vi "Audio Test.vi"() -> ()   [LabVIEW 2020, in "obs-scratch.lvlib"]
uses:
  obs-scratch.lvlib
  g-audio/src/LabVIEW/G-Audio/Controls/Audio Device Config.ctl
  g-audio/src/LabVIEW/G-Audio/Controls/Audio Device Format.ctl
  g-audio/src/LabVIEW/G-Audio/Controls/Backends.ctl
  g-audio/src/LabVIEW/G-Audio/Controls/Audio Device Info.ctl
  g-audio/src/LabVIEW/G-Audio/Controls/Audio Device Type.ctl
  g-audio/src/LabVIEW/G-Audio/Controls/Audio Device Native Data Format.ctl
  93cf9091-5c46-455b-b0da-0cb22890f002.vi
  <vilib>/Analysis/5stat.llb/RMS (DBL).vi
  g-audio/src/LabVIEW/G-Audio/Private/Result To Error.vi
  93cf9091-5c46-455b-b0da-0cb22890f002.vi/6b901882-6109-4f44-aca5-48e1525e5248.vi
  93cf9091-5c46-455b-b0da-0cb22890f002.vi/06c0137a-63d3-4e30-982f-115d83a1188c.vi
  g-audio/src/LabVIEW/G-Audio/Audio Devices/Get Audio Device Configuration.vi
  g-audio/src/LabVIEW/G-Audio/Private/Audio Device Refnum To Value.vi
  93cf9091-5c46-455b-b0da-0cb22890f002.vi/06c0137a-63d3-4e30-982f-115d83a1188c.vi/4b7b629c-2e91-4160-9820-a26af8f6e677.vi
  g-audio/src/LabVIEW/G-Audio/Private/ma_format To Audio Data Format.vi
  <vilib>/Utility/Data Type/Get Numeric Information.vi
  <vilib>/Utility/error.llb/Error Cluster From Error Code.vi
  g-audio/src/LabVIEW/G-Audio/G-Audio.lvlib
  <vilib>/Analysis/NI_AALPro.lvlib
  obs-websocket/OBS/OBS.lvclass
panel:
  in  "Gain":dbl
  in  "Scale Decay":dbl(slide) scale=0.0..1.0
  out "Scale":dbl(knob) scale=0.8..1.2
  in  "Password":string="44S4aN6PpCHpVM4Y"
  out "Meter":dbl(knob) scale=0.8..1.2
  out "error out":errorcluster
  in  "stop":bool
  out "Waveform":waveform(dbl)[](graph)
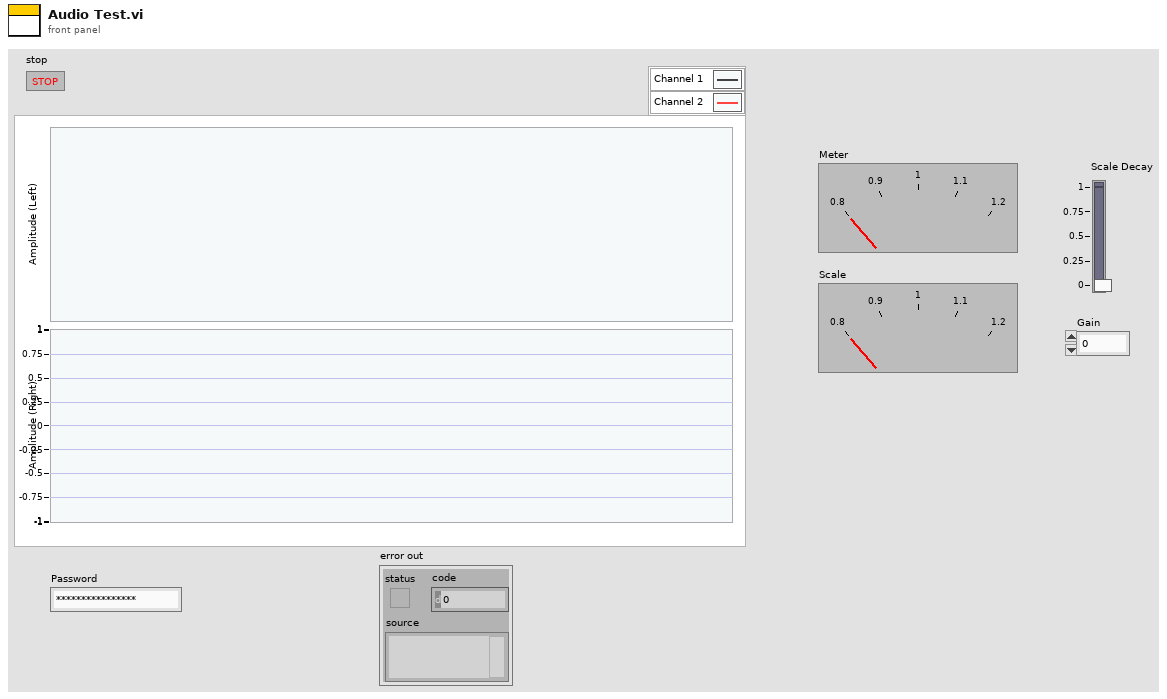
[diagram p1: front panel]
types:
  T1 = typedef "G-Audio.lvlib/Audio Device Type.ctl" = enum16{"(None)", "Playback", "Capture", "Duplex", "Loopback"}
  T2 = typedef "G-Audio.lvlib/Audio Device Info.ctl" = cluster{"Name":string, "ID":u8[], "Device Type":T1, "Default":bool, "Native Data Formats":T3[]}
  T3 = typedef "G-Audio.lvlib/Audio Device Native Data Format.ctl" = cluster{"Format":T4, "Channels":u32, "Sample Rate (Hz)":u32, "Exclusive Mode":bool}
  T4 = typedef "G-Audio.lvlib/Audio Device Format.ctl" = enum16{"Native", "U8", "I16", "I32", "SGL"}
  T5 = typedef "G-Audio.lvlib/Backends.ctl" = enum16{"WASAPI", "DirectSound", "WinMM", "Core Audio", "sndio", "audio(4)", "OSS", "PulseAudio", "ALSA", "JACK", "AAudio", "OpenSL|ES", "Web Audio", "Custom", "Null", "Default"}
  T6 = typedef "G-Audio.lvlib/Audio Device Config.ctl" = cluster{"Sample Rate (Hz)":u32, "Channels":u32, "Format":T4}
  T7 = typedef "G-Audio.lvlib/Audio Device Refnum.ctl" = refnum<file>
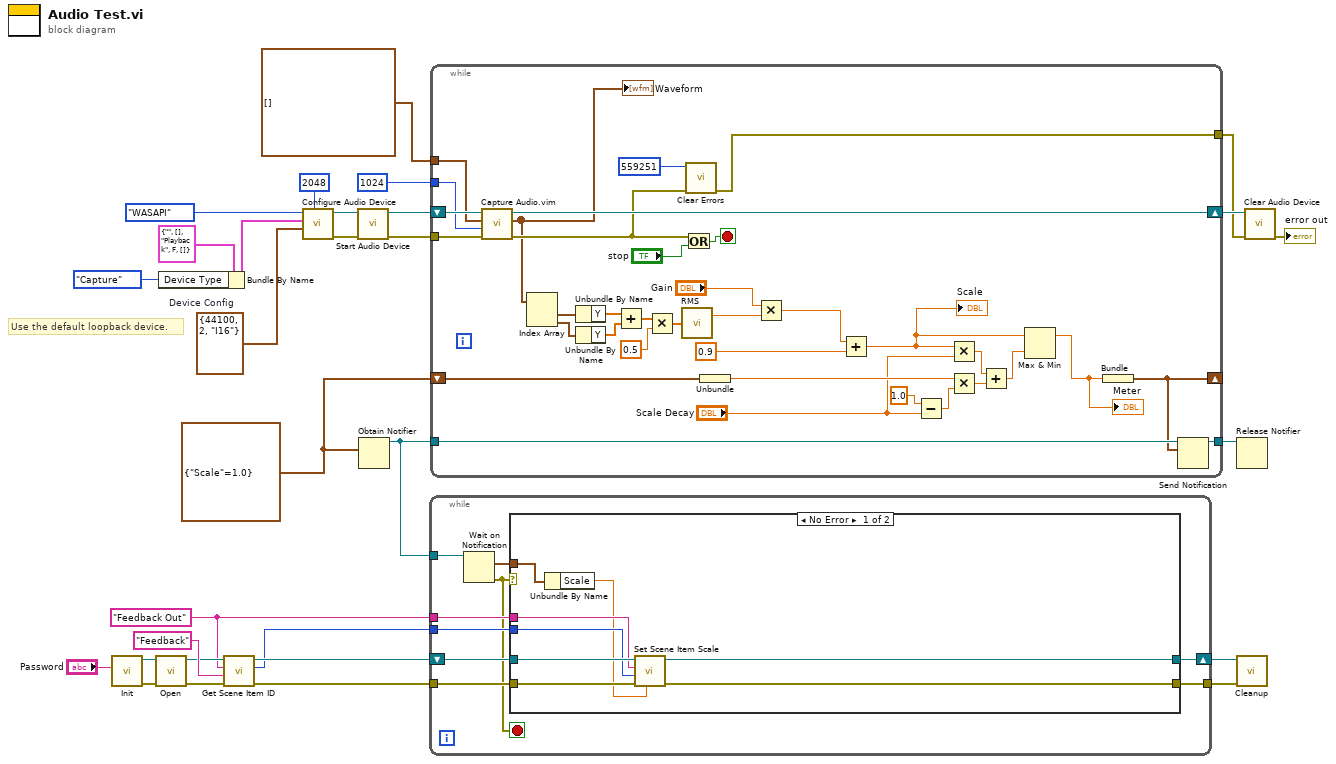
[diagram p0: block diagram]
diagram:
  w1 = cluster{"Scale":dbl} {"Scale"=1.0}
  w5 = "Feedback Out" ("Scene Name")
  w27 = T6 {"Sample Rate (Hz)"=44100, "Channels"=2, "Format"=enum."I16"}  # Device Config
  # "Use the default loopback device."
  n1 = call "Init.vi"("Password (None)"="Password") -> ("error out"=w14:errorcluster, "OBS out"=w15:refnum<class "OBS.lvclass">)  [unwired: 9 in]
  n2 = call "Open.vi"("error in (no error)"=w14, "OBS in"=w15) -> ("error out"=w10:errorcluster, "OBS out"=w11:refnum<class "OBS.lvclass">)  [unwired: 8 in]
  n3 = Bundle By Name(cluster=T2 {"Name"="", "ID"=[], "Device Type"=enum."Playback", "Default"=FALSE, "Native Data Formats"=[]} ("Audio Device"), "Device Type"=Audio_Device_Type."Capture") -> (w23:T2)
  n4 = call "Get Scene Item ID.vi"("error in (no error)"=w10, "Source Name"="Feedback" ("Scene Name"), "Scene Name"=w5, "OBS in"=w11) -> ("error out"=w9:errorcluster, "Scene Item ID"=w4:i32, "OBS out"=w8:refnum<class "OBS.lvclass">)  [unwired: 5 in]
  n5 = call "Configure Audio Device.vi"("Buffer Size (4096)"=2048 ("number of samples/ch"), "Device Config"=w27, "Audio Device"=w23, "Backend (Default)"=Backends."WASAPI") -> ("error out"=w30:errorcluster, "Audio Device Refnum"=w29:T7)  [unwired: 4 in, 2 out]
  n6 = call "Start Audio Device.vi"("error in (no error)"=w30, "Audio Device Refnum In"=w29) -> ("error out"=w22:errorcluster, "Audio Device Refnum Out"=w20:T7)  [unwired: 8 in]
  n7 = Obtain Notifier(notification data type=w1) -> (notifier out=w3:refnum<notifier>)  [unwired: 3 in, 2 out]
  n8 = while {
    tunnel: w9 -> [w36]
    shift-right: [w38] -> w7
    shift-left: w8 -> [w39]
    tunnel: [w37] -> w6
    tunnel: w5 -> [w35]
    tunnel: w4 -> [w34]
    tunnel: w3 -> [w33]
    stop <- w32 stop-if-true
    n9 = Wait on Notification(notifier=w33) -> (notification=w31:cluster{"Scale":dbl}, error out=w32:errorcluster)  [unwired: 3 in, 2 out]
    n10 = case shown="No Error" w32 {
      tunnel: w39 -> [w47 w49]
      tunnel: [w46 w49] -> w38
      tunnel: [w45 w48] -> w37
      tunnel: w36 -> [w44 w48]
      tunnel: w35 -> [w43 _]
      tunnel: w34 -> [w42 _]
      tunnel: w31 -> [w41 _]
      frame No Error {
        n11 = Unbundle By Name(w41) -> ("Scale"=w40:dbl)
        n12 = call "Set Scene Item Scale.vi"("Scale"=w40, "error in (no error)"=w44, "Scene Item ID"=w42, "Scene Name"=w43, "OBS in"=w47) -> ("error out"=w45:errorcluster, "OBS out"=w46:refnum<class "OBS.lvclass">)  [unwired: 5 in]
      }
      frame Error {
      }
    }
  }
  n13 = while {
    shift-right: [w83] -> w19
    shift-left: w20 -> [w84]
    tunnel: w22 -> [w81]
    tunnel: [w80] -> w18
    tunnel: 1024 ("number of samples/ch") -> [w75]
    tunnel: waveform(dbl)[] [] -> [w82]
    tunnel: w3 -> [w64]
    tunnel: [w63] -> w2
    shift-right: [w55] -> _
    shift-left: w1 -> [w62]
    stop <- w77 stop-if-true
    n14 = call "Capture Audio.vim"("error in (no error)"=w81, "Samples To Read"=w75, "Data Format"=w82, "Audio Device Refnum In"=w84) -> ("error out"=w78:errorcluster, "Audio Data"=w74:waveform(dbl)[], "Audio Device Refnum Out"=w83:T7)  [unwired: 5 in]
    "Waveform" <- w74
    n15 = Index Array(array=w74) -> (element #1=w73:waveform(dbl), element #2=w72:waveform(dbl))  [unwired: 2 in]
    n16 = Unbundle By Name(w73) -> ("Y"=w71:dbl[])
    n17 = Unbundle By Name(w72) -> ("Y"=w70:dbl[])
    n18 = Add(x=w71, y=w70) -> (x+y=w69:dbl[])
    n19 = Multiply(x=w69, y=0.5) -> (x*y=w67:dbl[])
    n20 = call-poly <vilib>:"RMS.vi"("X"=w67) -> ("rms value"=w66:dbl)  [unwired: 1 out]
    n21 = Or(x=w78, y="stop") -> (x .or. y?=w77:bool)
    n22 = call <vilib>:"Clear Errors.vi"("error in (no error)"=w78, "specific error code to clear (0: all)"=559251) -> ("error out"=w80:errorcluster)  [unwired: 4 in, 1 out]
    n23 = Unbundle(w62) -> ("Scale"=w60:dbl)
    n24 = Multiply(x="Gain", y=w66) -> (x*y=w51:dbl)
    n25 = Add(x=w51, y=0.9) -> (x+y=w54:dbl)
    "Scale" <- w54
    n26 = Subtract(x=1.0, y="Scale Decay") -> (x-y=w59:dbl)
    n27 = Multiply(x=w54, y="Scale Decay") -> (x*y=w56:dbl)
    n28 = Multiply(x=w60, y=w59) -> (x*y=w57:dbl)
    n29 = Add(x=w56, y=w57) -> (x+y=w53:dbl)
    n30 = Max & Min(x=w54, y=w53) -> (max(x,y)=w52:dbl)  [unwired: 1 out]
    "Meter" <- w52
    n31 = Bundle(w52) -> (w55:cluster{dbl})  [unwired: 1 in]
    n32 = Send Notification(notification=w55, notifier=w64) -> (notifier out=w63:refnum<notifier>)  [unwired: 1 in, 1 out]
  }
  n33 = Release Notifier(notifier=w2) -> ()  [unwired: 2 in, 3 out]
  n34 = call "Cleanup.vi"("error in (no error)"=w6, "OBS in"=w7) -> ()  [unwired: 9 in, 1 out]
  n35 = call "Clear Audio Device.vi"("error in (no error)"=w18, "Audio Device Refnum In"=w19) -> ("error out"=→"error out":errorcluster)  [unwired: 9 in]
